vi "Del Exp.vi"(8 "error in (no error)":errorcluster, 11 "Control-Client in":refnum<class "Control-Client.lvclass">) -> (0 "error out":errorcluster, 3 "Control-Client out":refnum<class "Control-Client.lvclass">)   [LabVIEW 2015, in "Control-Client.lvclass"]
uses:
  Control-Client.lvclass
  Control-Client.lvclass/Control-Client.ctl
  methods/Read Group #.vi
  Experiments/Experiments_group.lvclass
  Experiments/Experiment.lvclass
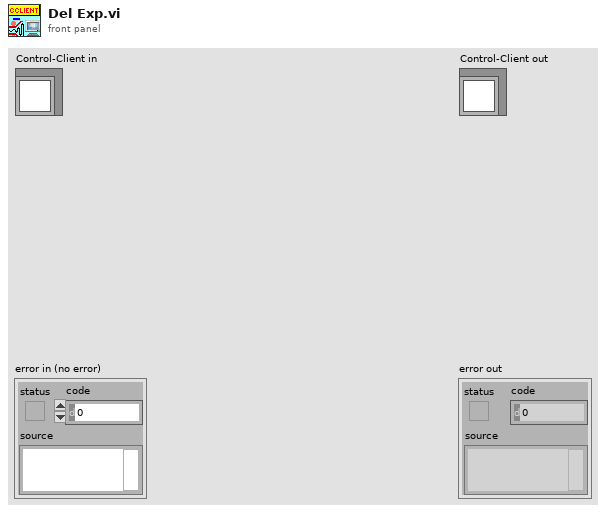
[diagram p1: front panel]
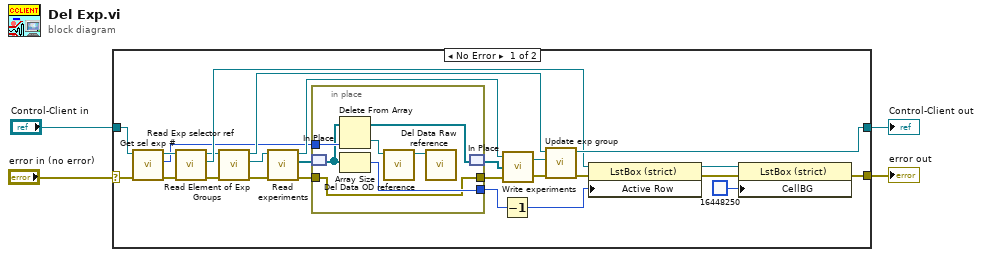
[diagram p0: block diagram]
diagram:
  n1 = case shown="No Error" "error in (no error)" {
    selector: "error in (no error)" -> [w28 w39]
    tunnel: [w13 w39] -> w3
    tunnel: [w20 w38] -> w1
    tunnel: "Control-Client in" -> [w25 w38]
    frame No Error {
      n2 = call "Get sel exp #.vi"("error in (no error)"=w28, "Control-Client in"=w25) -> ("error out"=w29:errorcluster, "Exp sel #"=w9:i32, "Control-Client out"=w27:refnum<class "Control-Client.lvclass">)  [unwired: 7 in]
      n3 = call "Read Exp selector ref.vi"("error in (no error)"=w29, "Control-Client in"=w27) -> ("error out"=w19:errorcluster, "Exp selector ref"=w18:refnum<vi>, "Control-Client out"=w6:refnum<class "Control-Client.lvclass">)  [unwired: 7 in]
      n4 = call "Read Element of Exp Groups.vi"("error in (no error)"=w19, "Control-Client in"=w6) -> ("error out"=w26:errorcluster, "Experiments_group.lvclass"=w24:refnum<class "Experiments_group.lvclass">, "Control-Client out"=w23:refnum<class "Control-Client.lvclass">)  [unwired: 7 in]
      n5 = call "Read experiments.vi"("error in (no error)"=w26, "Experiments_group.lvclass in"=w24) -> ("error out"=w8:errorcluster, "Experiments"=w11:refnum<class "Experiment.lvclass">[], "Experiments_group.lvclass out"=w12:refnum<class "Experiments_group.lvclass">)  [unwired: 6 in]
      n6 = in-place {
        in-place-border: w9 -> [w37]
        in-place-border: w8 -> [w31]
        in-place-border: [w31] -> w7
        in-place-border: [w32] -> w5
        n7 = in-place-match #1(w11) -> (w33:refnum<class "Experiment.lvclass">[])
        n8 = Delete From Array(array=w33, index=w37) -> (deleted portion=w34:refnum<class "Experiment.lvclass">, array with subset deleted=w36:refnum<class "Experiment.lvclass">[])  [unwired: 1 in]
        n9 = Array Size(array=w33) -> (size(s)=w32:i32)
        n10 = call "Del Data OD reference.vi"("Experiment in"=w34) -> ("Experiment out"=w35:refnum<class "Experiment.lvclass">)  [unwired: 9 in, 1 out]
        n11 = call "Del Data Raw reference.vi"("Experiment in"=w35) -> ()  [unwired: 9 in, 2 out]
        n12 = in-place-match #1(w36) -> (w10:refnum<class "Experiment.lvclass">[])
      }
      n13 = Decrement(x=w5) -> (x-1=w16:i32)
      n14 = call-dynamic "Write experiments.vi"("error in (no error)"=w7, "Experiments"=w10, "Experiments_group.lvclass in"=w12) -> ("error out"=w22:errorcluster, "Experiments_group.lvclass out"=w21:refnum<class "Experiments_group.lvclass">)
      n15 = call "Update exp group.vi"("error in (no error)"=w22, "Experiments_group.lvclass out"=w21, "Control-Client in"=w23) -> ("error out"=w14:errorcluster, "Control-Client out"=w20:refnum<class "Control-Client.lvclass">)  [unwired: 7 in]
      n16 = property on="Property Node" class="LstBox (strict)"(reference=w18, error in=w14, "Active Row"=w16) -> (reference out=w17:refnum<vi>, error out=w15:errorcluster)
      n17 = property on="Property Node" class="LstBox (strict)"(reference=w17, error in=w15, "CellBG"=u32 16448250) -> (error out=w13:errorcluster)  [unwired: 1 out]
    }
    frame Error {
    }
  }
  "error out" <- w3
  "Control-Client out" <- w1
